vi "FRCts20_WebMethods_ReadData_Team.vi"(7 "Team":T1, 8 "error in (no error)":errorcluster, 11 "httpRequestID":u32) -> (0 "error out":errorcluster, 2 "Team Out":T1, 3 "httpRequestID out":u32)   [LabVIEW 2013, in "FRCts20_WebMethods.lvlib"]
uses:
  FRCts20_WebMethods.lvlib
  <vilib>/wsapi/NI_WebServices.lvlib
  Backend/source/VI Source/FRCts20_Backend_Engine.lvlib
  <userlib>/_OpenG.lib/error/error.llb/Filter Error Codes (Array)__ogtk.vi
  Backend/source/VI Source/FRCts20_Backend_API/FRCts20_Backend_API_Status.ctl
  Backend/source/VI Source/FRCts20_Backend_API/FRCts20_Backend_API.lvlib
  Backend/source/VI Source/FRCts20_Backend_API/FRCts20_Backend_API_SW.ctl
  Backend/source/VI Source/FRCts20_Backend_API/FRCts20_Backend_API_Team.ctl
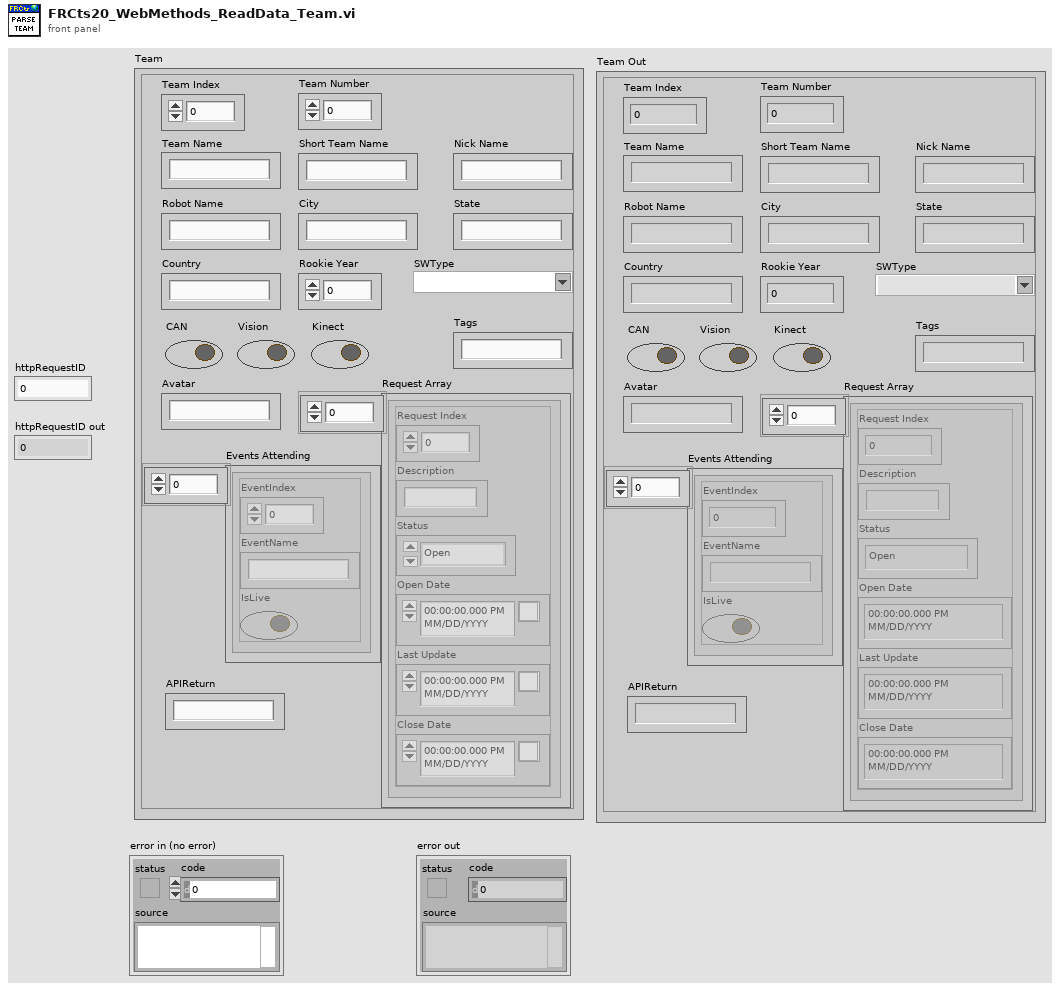
[diagram p1: front panel]
types:
  T1 = typedef "FRCts20_Backend_API.lvlib/FRCts20_Backend_API_Team.ctl" = cluster{"Team Index":u32, "Team Number":u32, "Team Name":string, "Short Team Name":string, "Nick Name":string, "Robot Name":string, "City":string, "State":string, "Country":string, "Rookie Year":u32, "SWType":T2, "CAN":bool, "Vision":bool, "Kinect":bool, "Tags":string, "Avatar":string, "Request Array":cluster{"Request Index":u32, "Description":string, "Status":T3, "Open Date":timestamp, "Last Update":timestamp, "Close Date":timestamp}[], "Events Attending":cluster{"EventIndex":dbl, "EventName":string, "IsLive":bool}[], "APIReturn":string}
  T2 = typedef "FRCts20_Backend_API.lvlib/FRCts20_Backend_API_SW.ctl" = string
  T3 = typedef "FRCts20_Backend_API.lvlib/FRCts20_Backend_API_Status.ctl" = enum16{"Open", "In Work", "Closed"}
  T4 = typedef "FRCts20_WebMethods.lvlib/FRCts20_WebMethods_ctl_returntype.ctl" = string
  T5 = cluster{"Local File Path":string, "Client File Name":string, "Content Type":string, "Size":u32}[]
  T6 = cluster{"Local File Path":string, "Client File Name":string, "Content Type":string, "Size":u32}
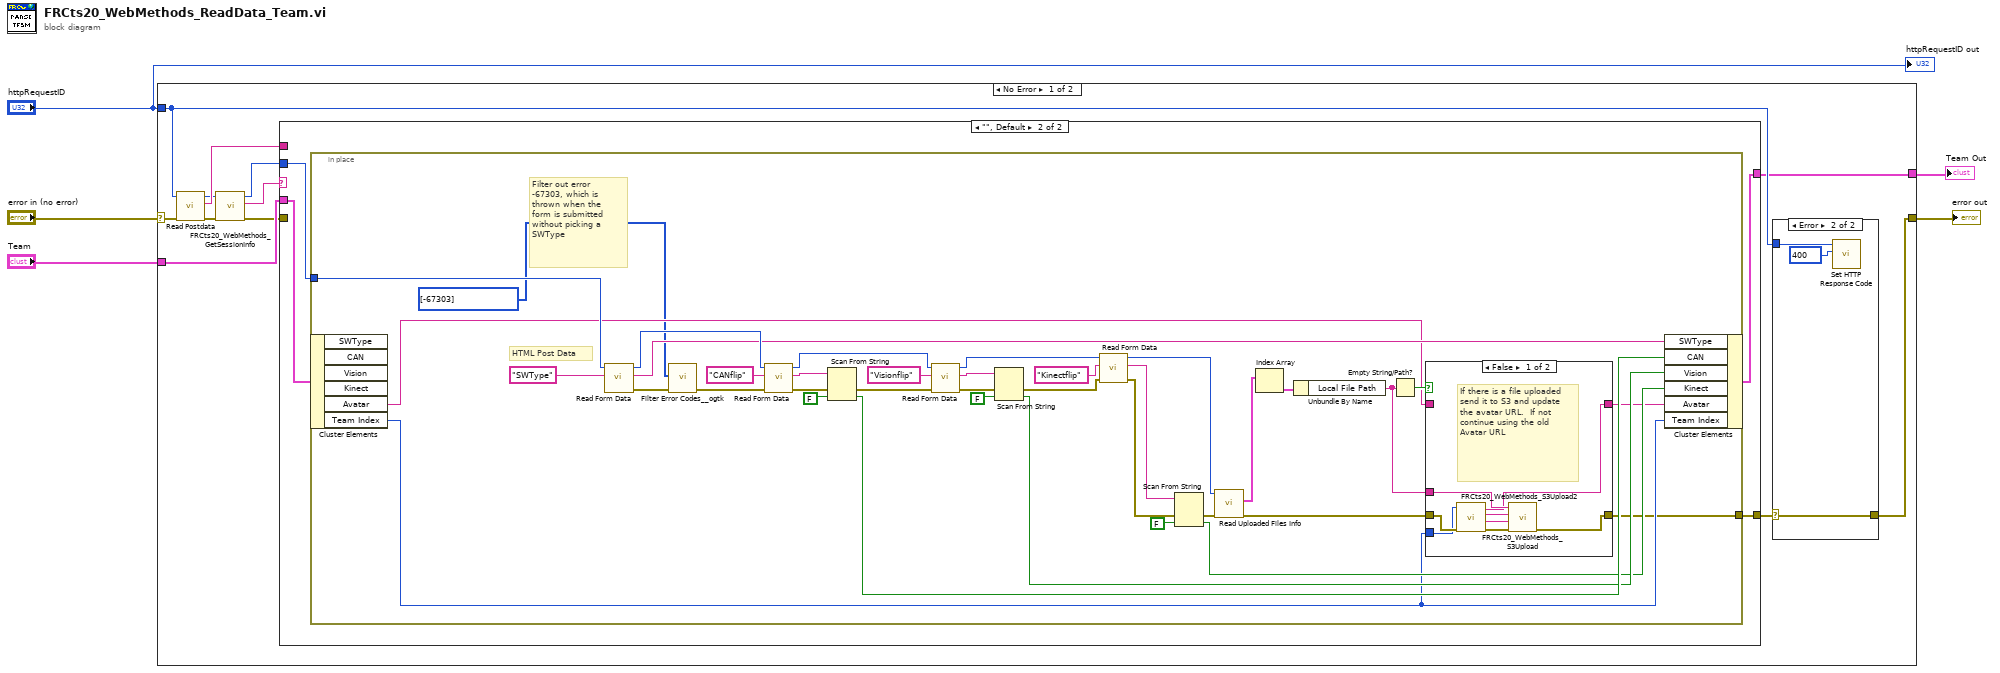
[diagram p0: block diagram]
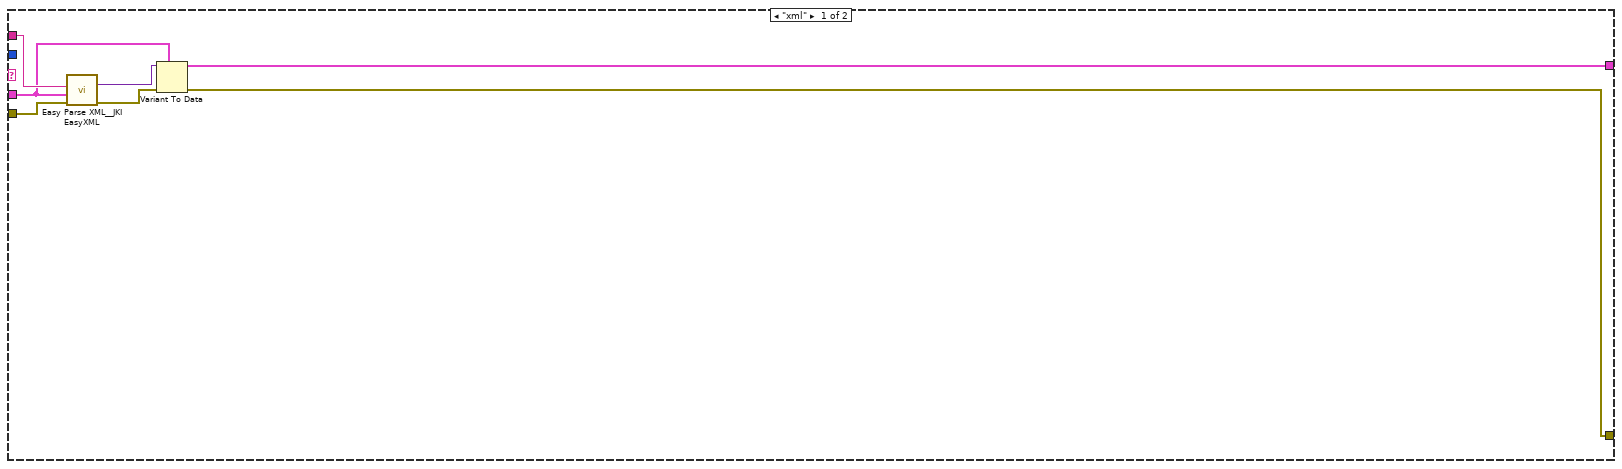
[diagram p2: hidden frame]
diagram:
  n1 = case shown="No Error" "error in (no error)" {
    selector: "error in (no error)" -> [w14 w81]
    tunnel: "httpRequestID" -> [w10 _]
    tunnel: "Team" -> [w16 w80]
    tunnel: [w15 w81] -> w4
    tunnel: [w6 w80] -> w1
    frame No Error {
      n2 = call <vilib>:"Read Postdata.vi"("error in (no error)"=w14, "httpRequestID"=w10) -> ("error out"=w13:errorcluster, "postdata"=w17:string, "httpRequestID out"=w9:u32)  [unwired: 7 in]
      n3 = call "FRCts20_WebMethods_GetSessionInfo.vi"("error in"=w13, "httpRequestID"=w9) -> ("error out"=w12:errorcluster, "Return Type"=w11:T4, "httpRequestID out"=w8:u32)  [unwired: 7 in]
      n4 = case shown="\"\", Default" w11 {
        tunnel: [w23 w28] -> w7
        tunnel: w16 -> [w19 w27]
        tunnel: [w18 w26] -> w6
        tunnel: w8 -> [_ w25]
        tunnel: w12 -> [w21 _]
        tunnel: w17 -> [w20 _]
        frame "xml" {
          n5 = call <vilib>:"Easy Parse XML__JKI EasyXML.vi"("error in (no error)"=w21, "LabVIEW Data (Type)"=w19, "XML String"=w20) -> ("error out"=w22:errorcluster, "LabVIEW Data"=w24:variant)  [unwired: 7 in]
          n6 = Variant To Data(error in=w22, type=w19, Variant=w24) -> (data=w18:T1, error out=w23:errorcluster)
        }
        frame "", Default {
          n7 = in-place {
            in-place-border: w25 -> [w65]
            in-place-border: [w39] -> w28
            # "Filter out error -67303, which is thrown when the form is submitted without picking a SWType"
            # "HTML Post Data"
            n8 = in-place-cluster #1(w27) -> ("Avatar"=w32:string, "Team Index"=w40:u32)  [unwired: 4 out]
            n9 = call <vilib>:"Read Form Data.vi"("key"="SWType", "httpRequestID"=w65) -> ("error out"=w31:errorcluster, "value"=w43:string, "httpRequestID out"=w64:u32)  [unwired: 6 in, 1 out]
            n10 = call-poly <userlib>:"Filter Error Codes__ogtk.vi"("Error In"=w31, "Error Codes to Filter"=i32[] [-67303]) -> ("Error Out"=w30:errorcluster)  [unwired: 7 in, 2 out]
            n11 = call <vilib>:"Read Form Data.vi"("error in (no error)"=w30, "key"="CANflip", "httpRequestID"=w64) -> ("error out"=w56:errorcluster, "value"=w54:string, "httpRequestID out"=w61:u32)  [unwired: 5 in, 1 out]
            n12 = Scan From String(input string=w54, error in=w56, default 1=FALSE) -> (error out=w55:errorcluster, output 1=w46:bool)  [unwired: 2 in, 2 out]
            n13 = call <vilib>:"Read Form Data.vi"("error in (no error)"=w55, "key"="Visionflip", "httpRequestID"=w61) -> ("error out"=w53:errorcluster, "value"=w51:string, "httpRequestID out"=w59:u32)  [unwired: 5 in, 1 out]
            n14 = Scan From String(input string=w51, error in=w53, default 1=FALSE) -> (error out=w52:errorcluster, output 1=w45:bool)  [unwired: 2 in, 2 out]
            n15 = call <vilib>:"Read Form Data.vi"("error in (no error)"=w52, "key"="Kinectflip", "httpRequestID"=w59) -> ("error out"=w49:errorcluster, "value"=w48:string, "httpRequestID out"=w37:u32)  [unwired: 5 in, 1 out]
            n16 = Scan From String(input string=w48, error in=w49, default 1=FALSE) -> (error out=w38:errorcluster, output 1=w44:bool)  [unwired: 2 in, 2 out]
            n17 = call <vilib>:"Read Uploaded Files Info.vi"("error in (no error)"=w38, "httpRequestID"=w37) -> ("error out"=w41:errorcluster, "UploadedFilesList"=w36:T5)  [unwired: 7 in, 1 out]
            n18 = Index Array(array=w36) -> (element=w42:T6)  [unwired: 1 in]
            n19 = Unbundle By Name(w42) -> ("Local File Path"=w34:string)
            n20 = Empty String/Path?(string/path=w34) -> (empty?=w35:bool)
            n21 = case shown="False" w35 {
              tunnel: w41 -> [w73 w74]
              tunnel: w40 -> [w72 _]
              tunnel: [w71 w74] -> w39
              tunnel: w34 -> [w67 _]
              tunnel: [w66 w75] -> w33
              tunnel: w32 -> [_ w75]
              frame False {
                # "If there is a file uploaded send it to S3 and update the avatar URL.  If not continue using the old Avatar URL"
                n22 = call "FRCts20_WebMethods_S3Upload2.vi"("error in (no error)"=w73, "Team Index"=w72) -> ("error out"=w68:errorcluster, "Bucket"=w69:string, "Object Path"=w70:string, "S3 URL"=w66:string)  [unwired: 6 in]
                n23 = call "FRCts20_WebMethods_S3Upload.vi"("error in (no error)"=w68, "Bucket"=w69, "Object Path"=w70, "Temporary URL"=w67) -> ("error out"=w71:errorcluster)  [unwired: 7 in]
              }
              frame True {
              }
            }
            n24 = in-place-cluster #1("SWType"=w43, "CAN"=w46, "Vision"=w45, "Kinect"=w44, "Avatar"=w33, "Team Index"=w40) -> (w26:T1)
          }
        }
      }
      n25 = case shown="Error" w7 {
        selector: w7 -> [w76 w77]
        tunnel: [w76 w77] -> w15
        tunnel: w10 -> [_ w79]
        frame No Error {
        }
        frame Error {
          w78 = 400 items=["100"=100, "101"=101, "200"=200, "201"=201, "202"=202, "203"=203, "204"=204, "205"=205, "206"=206, "300"=300, "301"=301, "302"=302, "303"=303, "304"=304, "305"=305, "306"=306, "307"=307, "400"=400, "401"=401, "402"=402, "403"=403, "404"=404, "405"=405, "406"=406, "407"=407, "408"=408, "409"=409, "410"=410, "411"=411, "412"=412, "413"=413, "414"=414, "415"=415, "416"=416, "417"=417, "500"=500, "501"=501, "502"=502, "503"=503, "504"=504, "505"=505] ("response code (200)")
          n26 = call <vilib>:"Set HTTP Response Code.vi"("response code (200)"=w78, "httpRequestID"=w79) -> ()  [unwired: 8 in, 2 out]
        }
      }
    }
    frame Error {
    }
  }
  "error out" <- w4
  "Team Out" <- w1
  "httpRequestID out" <- "httpRequestID"
